vi "G#RealTimeTemplate_GetAttributes.vi"(0 "reference in":refnum<class "G#RealTimeTemplate.lvclass">, 1 "return data? (T)":bool=TRUE, 5 "error in (no error)":errorcluster) -> (14 "reference out":refnum<class "G#RealTimeTemplate.lvclass">, 15 "attributes ref":T2, 16 "attributes":T1, 19 "error out":errorcluster)   [LabVIEW 2020, in "G#RealTimeTemplate.lvclass"]
doc: "Returns a reference and if wanted the actual data values of the attributes. This method is used by the subclasses to access parent attributes."
uses:
  <vilib>/addons/_AddQ/G#Templates/G#RealTimeTemplate/G#RealTimeTemplate.lvclass
  <vilib>/addons/_AddQ/G#Templates/G#RealTimeTemplate/utils/ObjectAttributesRef.ctl
  <vilib>/addons/_AddQ/G#Templates/G#RealTimeTemplate/protected/ObjectAttributes.ctl
  <vilib>/addons/_AddQ/G#Templates/G#RealTimeTemplate/G#RealTimeTemplate.lvclass/G#RealTimeTemplate.ctl
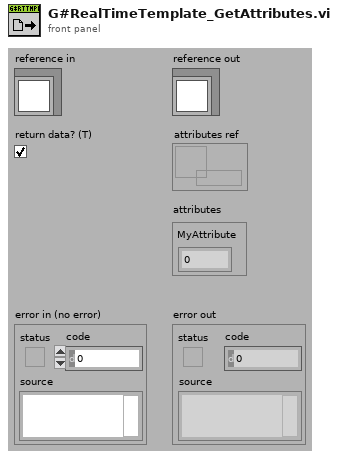
[diagram p1: front panel]
types:
  T1 = typedef "G#RealTimeTemplate.lvclass/ObjectAttributes.ctl" = cluster{"MyAttribute":dbl}
  T2 = typedef "G#RealTimeTemplate.lvclass/ObjectAttributesRef.ctl" = refnum<data-value>
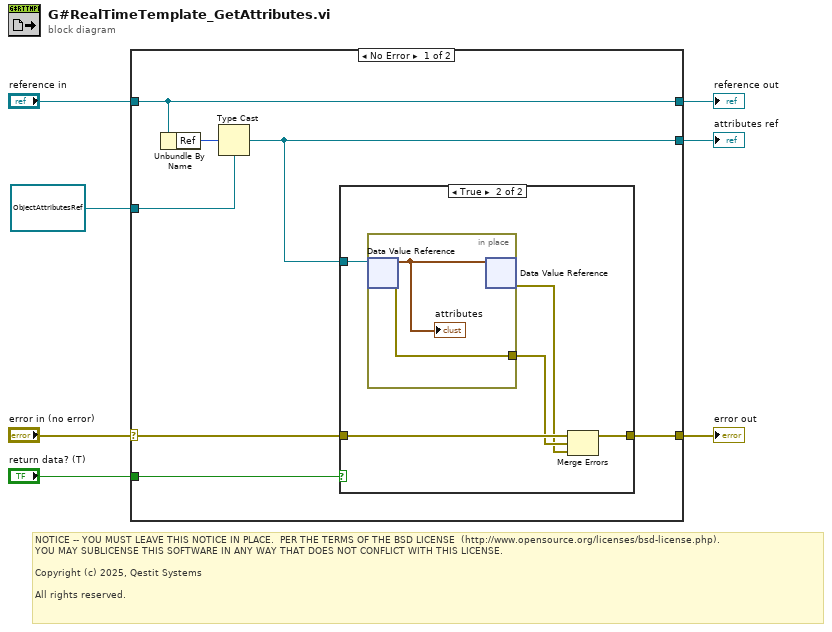
[diagram p0: block diagram]
diagram:
  # "NOTICE -- YOU MUST LEAVE THIS NOTICE IN PLACE.  PER THE TERMS OF THE BSD LICENSE  (http://www.opensource.org/licenses/bsd-license.php).\nYOU MAY SUBLICENSE THIS SOFTWARE IN ANY WAY THAT DOES NOT CONFLICT WITH THIS LICENSE.\n\nCopyright (c) 2025, Qestit Systems\n\nAll rights reserved."
  n1 = case shown="No Error" "error in (no error)" {
    selector: "error in (no error)" -> [w11 w25]
    tunnel: [w13 w25] -> w6
    tunnel: [w10 w24] -> w4
    tunnel: "reference in" -> [w10 w24]
    tunnel: [w8 w23] -> w3
    tunnel: "return data? (T)" -> [w14 _]
    tunnel: T2 refnum ("attributes ref") -> [w9 w23]
    frame No Error {
      n2 = Unbundle By Name(w10) -> ("Ref"=w12:u32)
      n3 = Type Cast(type=w9, x=w12) -> (*(type *) &x=w8:T2)
      n4 = case shown="True" w14 {
        tunnel: w8 -> [_ w20]
        tunnel: w11 -> [w15 w19]
        tunnel: [w15 w18] -> w13
        frame False {
        }
        frame True {
          n5 = in-place {
            in-place-border: [w22] -> w17
            n6 = in-place-dvr #1(w20) -> (w21:T1, w22:errorcluster)
            "attributes" <- w21
            n7 = in-place-dvr #1(w21) -> (w16:errorcluster)  [unwired: 1 out]
          }
          n8 = Merge Errors(w19, w17, w16) -> (w18:errorcluster)
        }
      }
    }
    frame Error {
    }
  }
  "error out" <- w6
  "reference out" <- w4
  "attributes ref" <- w3
